vi "氨氮质控流程.vi"(7 "队列输入NH3":refnum<queue>, 10 "氨氮":bool, 11 "氨氮量程切换":enum32{"H", "L", "AUTO"}(ring)=enum."AUTO") -> (2 "氨氮中断报警":bool, 3 "布尔":bool)   [LabVIEW 2016, in "质控单元.lvlib"]
uses:
  <vilib>/ptbypt/NI_PtbyPt.lvlib
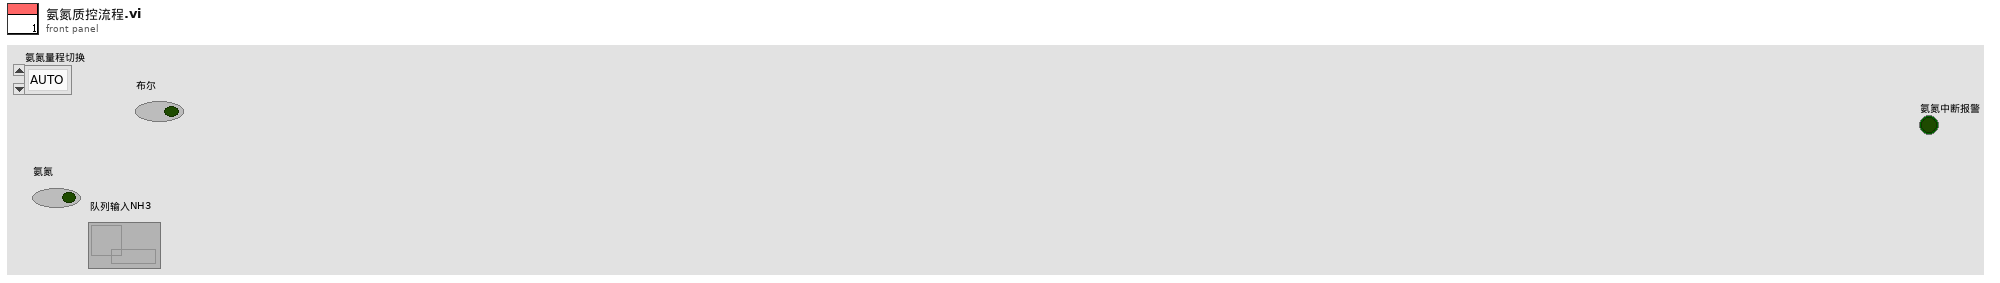
[diagram p1: front panel]
types:
  T1 = enum16{"待机", "启动氨氮水样", "氨氮测量中", "启动氨氮加标", "启动氨氮加标回收", "氨氮加标回收测量中", "启动总氮水样", "总氮测量中", "启动总氮加标", "启动总氮加标回收", "总氮加标回收测量中", "启动总磷水样", "总磷水样测量中", "启动总磷加标", "启动总磷加标回收", "总磷加标回收测量中", "结束"}
  T2 = cluster{"站号":u16, "量程切换":enum32{"H", "L", "AUTO"}, "控制命令":enum16{"启动测量", "标样核查", "零点核查", "跨度核查", "空白测试", "平行样测试", "加标回收", "空白校准", "标样校准", "初始化（清洗）", "停止测试", "仪器重启", "校时", "模式设置", "测量间隔设置"}, "模式设置":enum16{"待机", "连续模式", "周期模式", "定点模式", "受控模式", "手动模式"}, "测量间隔":u16}
  T3 = cluster{"时间标识":timestamp, "设备":string, "日志信息":string}
  T4 = cluster{"命令":string, cluster{"starting address":u16, "holding register value":u16}}
  T5 = cluster{"系统时间":timestamp, "工作状态":enum16{"空闲", "水样测试", "标样核查", "零点核查", "跨度核查", "空白测试", "平行样测试", "加标回收", "空白校准", "标样校准", "初始化（清洗）"}, "测量模式":enum16{"待机", "连续模式", "周期模式", "定点模式", "受控模式", "手动模式"}, "告警代码":enum16{"无告警", "缺试剂告警", "缺水样告警", "缺蒸馏水告警", "缺标液告警", "仪表漏液告警", "标定异常告警", "超量程告警", "加热异常", "低试剂预警", "超上限告警", "超下限告警", "仪表内部其他异常", "滴定异常告警", "电极异常告警", "量程切换告警", "参数设置告警", "PH电极电位异常", "电导率电极异常", "浊度光度异常", "溶解氧电极异常", "溶解氧光强异常", "温度异常告警", "PH异常告警", "溶解氧异常告警", "电导率异常告警", "浊度异常告警", "叶绿素异常告警", "藻密度异常告警", "蓝绿藻异常告警", "ORP异常告警", "氨氮异常告警", "清洁刷异常告警", "SD卡异常告警", "蓝牙异常告警", "Wifi异常告警", "流程异常告警"}, "故障代码":enum16{"无故障", "电机故障", "温度故障", "通讯故障", "滴定故障"}, "日志代码":u16, "软件版本":u16, "F0":sgl, "F1":sgl, "F2":sgl, "F3":sgl, "T":sgl, "H":sgl, "id":u16, "flowid":u16, "量程":u16, "总磷控温温度1":sgl, "营养盐控温温度2":sgl, "ADC":sgl}
  T6 = enum16{"空闲", "水样测试", "标样核查", "零点核查", "跨度核查", "空白测试", "平行样测试", "加标回收", "空白校准", "标样校准", "初始化（清洗）"}
  T7 = cluster{"因子编码":u32, "单位":u16, "标样参考值":sgl, "水样数据时间":timestamp, "水样实测值":sgl, "水样数据标识":string, "标样数据时间":timestamp, "标样实测值":sgl, "标样数据标识":string, "空白数据时间":timestamp, "空白实测值":sgl, "空白数据标识":string, "零点核查数据时间":timestamp, "零点核查实测值":sgl, "零点核查数据标识":string, "跨度核查数据时间":timestamp, "跨度核查实测值":sgl, "跨度核查数据标识":string, "加标回收数据时间":timestamp, "加标回收实测值":sgl, "加标回收数据标识":string, "平行样数据时间":timestamp, "平行样实测值":sgl, "平行样数据标识":string}
  T8 = cluster{"量程":dbl, "检出限":dbl, "加标前水样浓度":dbl, "加标后水样浓度":dbl, "加标水杯定容体积":dbl, "加标母液浓度":dbl, "加标体积":dbl, "加标回收率":dbl}
  T9 = cluster{"氨氮":u8, "总磷":u8, "总氮":u8, "CODMn":u8, "CODCr":u8}
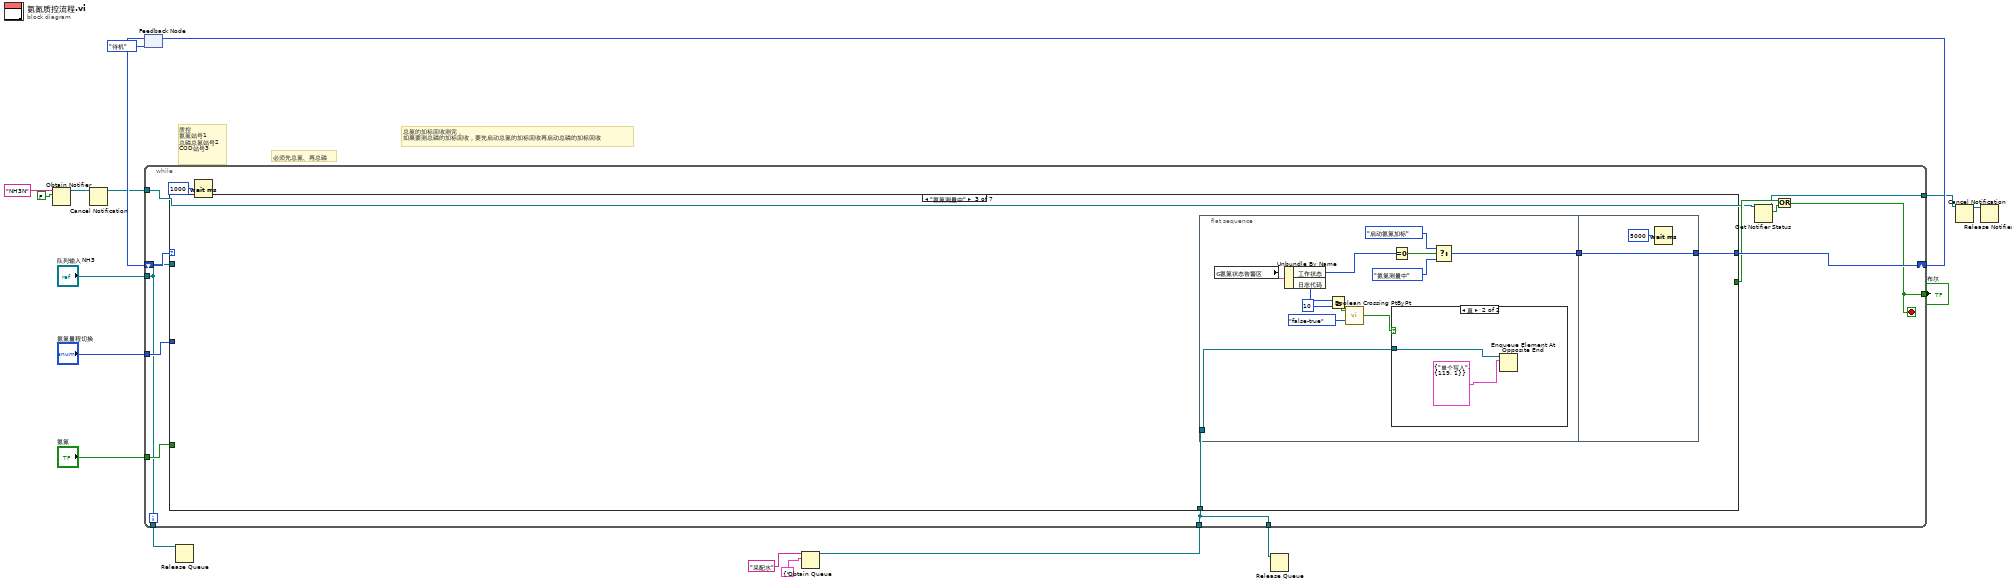
[diagram p0: block diagram]
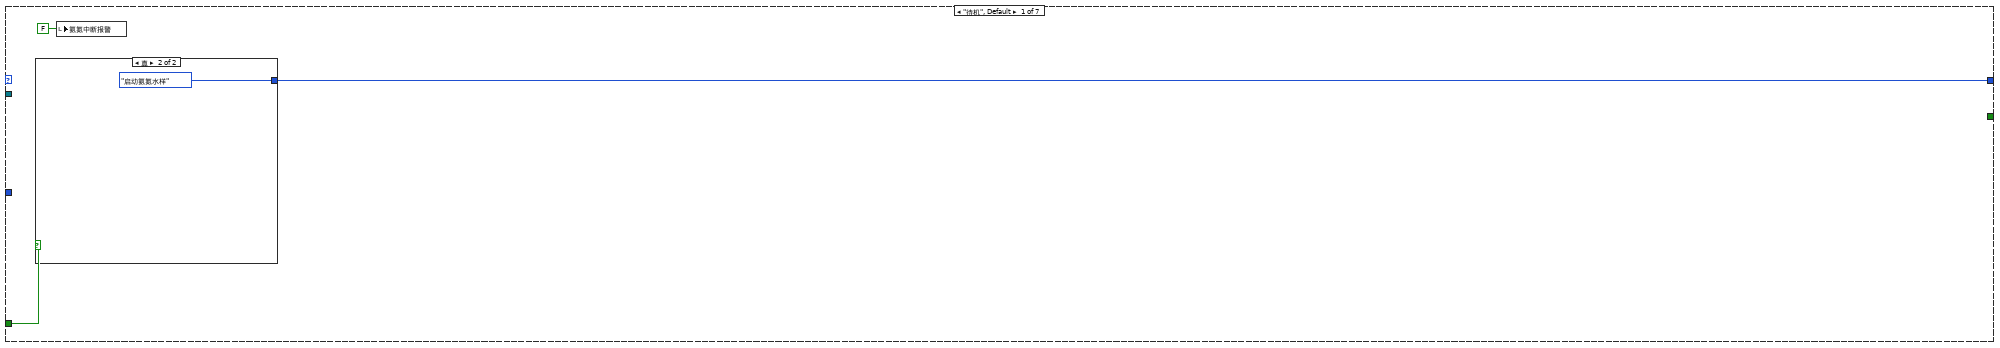
[diagram p2: hidden frame]
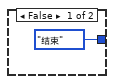
[diagram p3: hidden frame]
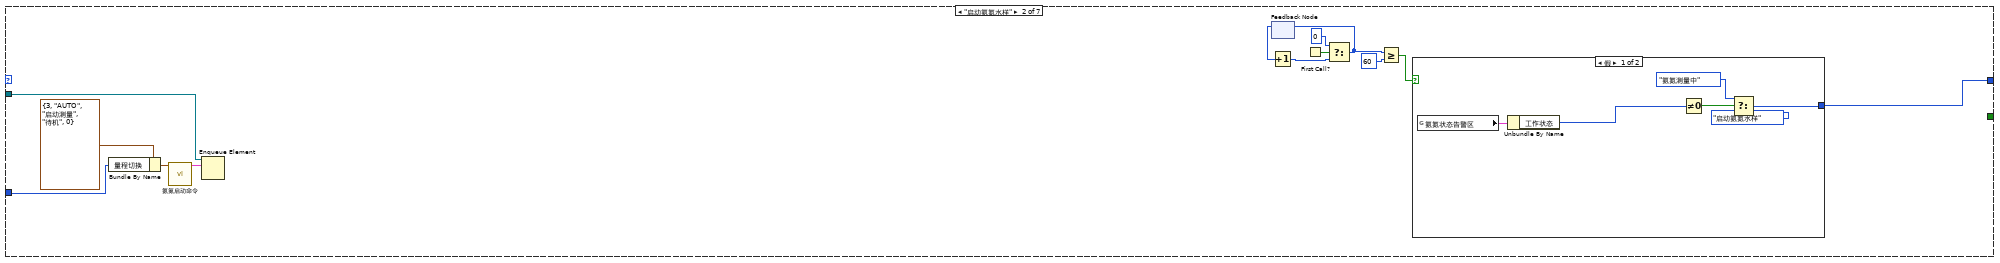
[diagram p4: hidden frame]
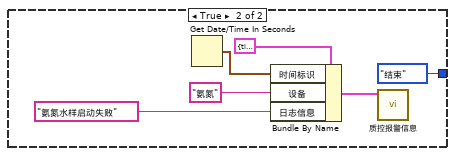
[diagram p5: hidden frame]
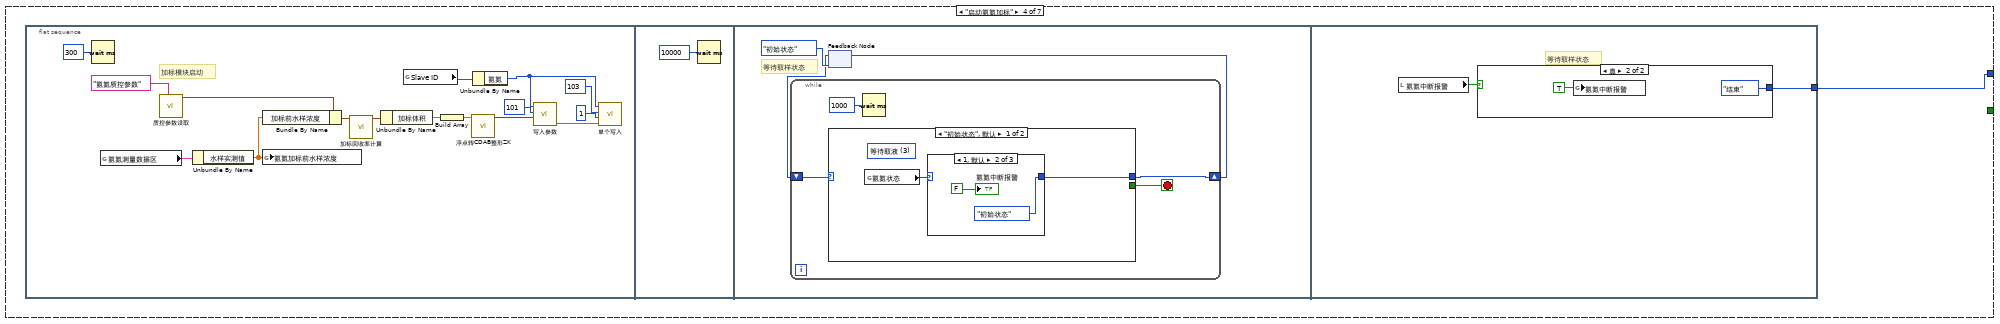
[diagram p7: hidden frame]
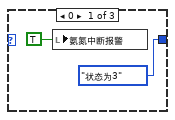
[diagram p8: hidden frame]
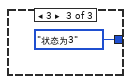
[diagram p9: hidden frame]
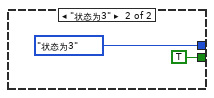
[diagram p10: hidden frame]
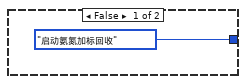
[diagram p11: hidden frame]
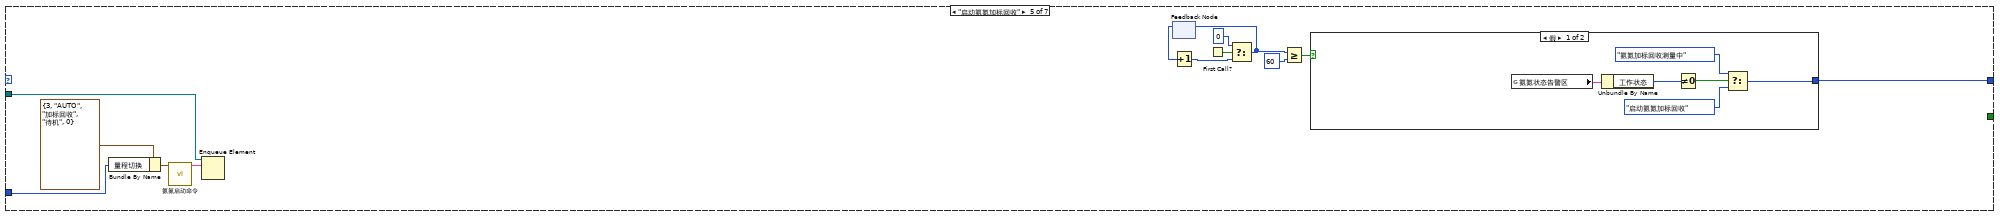
[diagram p12: hidden frame]
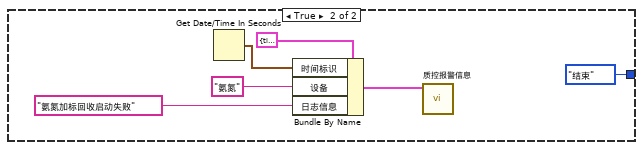
[diagram p13: hidden frame]
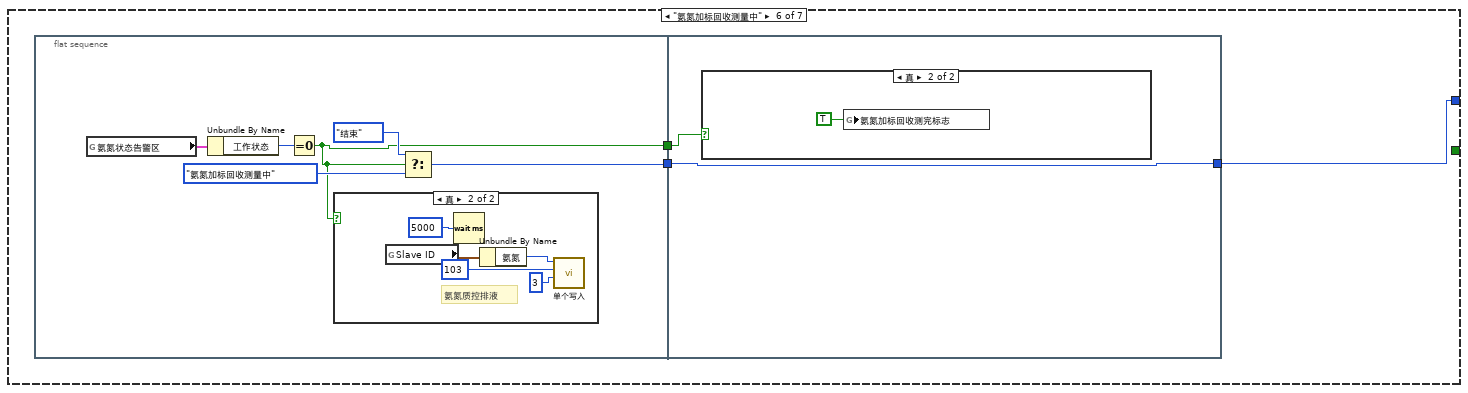
[diagram p14: hidden frame]
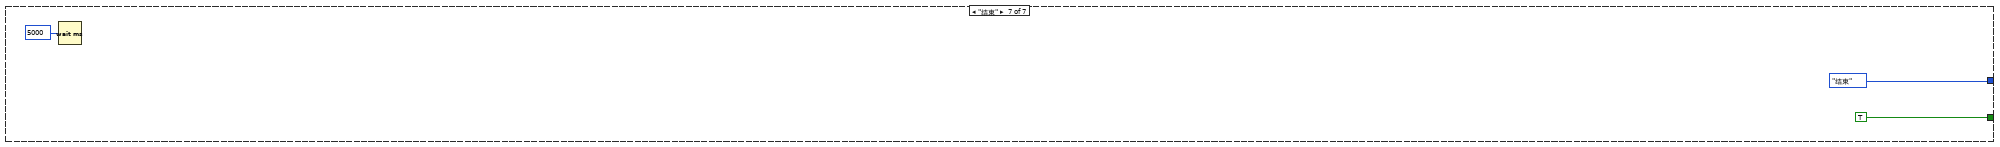
[diagram p17: hidden frame]
diagram:
  # "总氮的加标回收测完，\n如果要测总磷的加标回收，要先启动总氮的加标回收再启动总磷的加标回收"
  # "质控\n氨氮站号1   \n总磷总氮站号2\nCOD站号3"
  # "必须先总氮、再总磷"
  n1 = Obtain Notifier(name (unnamed)="NH3N" ("名称（未命名）"), notification data type=FALSE) -> (notifier out=w9:refnum<notifier>)  [unwired: 2 in, 2 out]
  n2 = Cancel Notification(0:w9) -> (8:w1:refnum<notifier>)  [unwired: 1 in, 2 out]
  n3 = feedback #1(T1."待机") -> (w12:T1)
  n4 = Obtain Queue(name (unnamed)="采配水" ("名称（未命名）"), element data type=cluster{"命令":string, "数据":variant} {"命令"="", "数据"=variant}) -> (queue out=w4:refnum<queue>)  [unwired: 3 in, 2 out]
  n5 = while {
    tunnel: "队列输入NH3" -> [w20]
    tunnel: "氨氮量程切换" -> [w28]
    tunnel: "氨氮" -> [w30]
    tunnel: [w23] -> w17
    shift-right: [w29] -> w15
    shift-left: w12 -> [w27]
    tunnel: w1 -> [w21]
    tunnel: [w22] -> w7
    tunnel: w4 -> [w19]
    tunnel: [w20] -> w3
    tunnel: [w19] -> w2
    stop <- w23 stop-if-true
    n6 = case shown="\"氨氮测量中\"" w27 {
      tunnel: [w33 w48 w63 w80 w124 w145 T1."结束"] -> w29
      tunnel: [_ _ _ _ _ _ TRUE] -> w24
      tunnel: w30 -> [w32 _ _ _ _ _ _]
      tunnel: w20 -> [_ w39 _ _ w122 _ _]
      tunnel: w28 -> [_ w36 _ _ w119 _ _]
      tunnel: w19 -> [_ _ w61 _ _ _ _]
      frame "待机", Default {
        n7 = case shown="真" w32 {
          tunnel: [T1."结束" T1."启动氨氮水样"] -> w33
          frame False {
          }
          frame True {
          }
        }
        n8 = local write "氨氮中断报警"(FALSE ("氨氮中断报警")) -> ()
      }
      frame "启动氨氮水样" {
        n9 = Bundle By Name(cluster=T2 {"站号"=3, "量程切换"=enum."AUTO", "控制命令"=enum."启动测量", "模式设置"=enum."待机", "测量间隔"=0} ("参数"), "量程切换"=w36) -> (w37:T2)
        n10 = call "氨氮启动命令.vi"("参数"=w37) -> ("启动命令"=w40:cluster{"命令":string, "data":variant})  [unwired: 10 in]
        n11 = Enqueue Element(queue=w39, element=w40) -> ()  [unwired: 2 in, 3 out]
        n12 = feedback #2() -> (w45:i32)  [unwired: 1 in]
        n13 = Increment(x=w45) -> (x+1=w44:i32)
        n14 = First Call?() -> (First Call?: T/F=w46:bool)
        n15 = Select(t=0, s=w46, f=w44) -> (s? t:f=w43:i32)
        n16 = feedback-in #2(w43) -> ()
        n17 = Greater Or Equal?(x=w43, y=60) -> (x >= y?=w41:bool)
        n18 = case shown="假" w41 {
          tunnel: [w52 T1."结束"] -> w48
          frame False {
            n19 = global read "与氨氮交互全局.vi" "氨氮状态告警区"() -> (w49:T5)
            n20 = Unbundle By Name(w49) -> ("工作状态"=w54:T6)
            n21 = Not Equal To 0?(x=w54) -> (x != 0?=w53:bool)
            n22 = Select(t=T1."氨氮测量中", s=w53, f=T1."启动氨氮水样") -> (s? t:f=w52:T1)
          }
          frame True {
            n23 = Get Date/Time In Seconds() -> (seconds since 1Jan1904=w60:timestamp)
            n24 = Bundle By Name(cluster=T3 {"时间标识"=timestamp(0 s since 1904-01-01), "设备"="", "日志信息"=""} ("data in"), "时间标识"=w60, "设备"="氨氮", "日志信息"="氨氮水样启动失败") -> (w55:T3)
            n25 = call "质控报警信息.vi"("data in"=w55) -> ()  [unwired: 11 in]
          }
        }
      }
      frame "氨氮测量中" {
        n26 = flat-sequence {
          tunnel: [w74] -> w62
          tunnel: w61 -> [w64]
          tunnel: [w79] -> w63
          tunnel: w62 -> [w79]
          frame #0 {
            n27 = global read "与氨氮交互全局.vi" "氨氮状态告警区"() -> (w70:T5)
            n28 = Unbundle By Name(w70) -> ("工作状态"=w75:T6, "日志代码"=w69:u16)
            n29 = Greater Or Equal?(x=w69, y=u16 10) -> (x >= y?=w67:bool)
            n30 = call <vilib>:"Boolean Crossing PtByPt.vi"("direction"=enum16{"either", "false-true", "true-false"}."false-true", "input"=w67) -> ("crossing"=w65:bool)  [unwired: 1 in]
            n31 = case shown="真" w65 {
              tunnel: w64 -> [_ w76]
              frame False {
              }
              frame True {
                n32 = Enqueue Element At Opposite End(queue=w76, element=T4 {"命令"="单个写入", {"starting address"=119, "holding register value"=1}} ("元素")) -> ()  [unwired: 2 in, 3 out]
              }
            }
            n33 = Equal To 0?(x=w75) -> (x = 0?=w73:bool)
            n34 = Select(t=T1."启动氨氮加标", s=w73, f=T1."氨氮测量中") -> (s? t:f=w74:T1)
          }
          frame #1 {
            n35 = Wait (ms)(milliseconds to wait=u32 5000 ("等待时间（毫秒）")) -> ()  [unwired: 1 out]
          }
        }
      }
      frame "启动氨氮加标" {
        n36 = flat-sequence {
          tunnel: [w115] -> w80
          frame #0 {
            # "加标模块启动"
            n37 = Wait (ms)(milliseconds to wait=u32 300 ("等待时间（毫秒）")) -> ()  [unwired: 1 out]
            n38 = global read "与氨氮交互全局.vi" "氨氮测量数据区"() -> (w84:T7)
            n39 = call "质控参数读取.vi"("section"="氨氮质控参数") -> ("参数"=w94:T8)  [unwired: 9 in, 1 out]
            n40 = Unbundle By Name(w84) -> ("水样实测值"=w85:sgl)
            n41 = Bundle By Name(cluster=w94, "加标前水样浓度"=w85) -> (w95:T8)
            n42 = global write "水样浓度全局.vi" "氨氮加标前水样浓度"(w85) -> ()
            n43 = call "加标回收率计算.vi"("参数"=w95) -> ("参数 out"=w93:T8)  [unwired: 9 in, 1 out]
            n44 = Unbundle By Name(w93) -> ("加标体积"=w86:dbl)
            n45 = global read "断电保存全局.vi" "Slave ID"() -> (w82:T9)
            n46 = Build Array(w86) -> (w92:dbl[])
            n47 = call "浮点转CDAB整形ZK.vi"("浮点数"=w92) -> ("CDAB整形输出"=w87:u16[])  [unwired: 10 in]
            n48 = Unbundle By Name(w82) -> ("氨氮"=w81:u8)
            n49 = call "写入参数.vi"("values"=w87, "starting address"=u16 101, "Slave ID"=w81) -> ("error out"=w91:errorcluster)  [unwired: 8 in]
            n50 = call "单个写入.vi"("Error in"=w91, "value"=u16 1, "address"=u16 103, "Slave ID"=w81) -> ()  [unwired: 7 in, 1 out]
          }
          frame #1 {
            n51 = Wait (ms)(milliseconds to wait=u32 10000 ("等待时间（毫秒）")) -> ()  [unwired: 1 out]
          }
          frame #2 {
            # "等待取样状态"
            n52 = feedback #3(enum16{"初始状态", "状态为3"}."初始状态") -> (w99:enum16{"初始状态", "状态为3"})
            n53 = while {
              shift-right: [w103] -> w98
              shift-left: w99 -> [w104]
              stop <- w102 stop-if-true
              n54 = case shown="\"初始状态\", 默认" w104 {
                tunnel: [w106 enum16{"初始状态", "状态为3"}."状态为3"] -> w103
                tunnel: [_ TRUE] -> w102
                frame "初始状态", Default {
                  (unwired) u16 3 items=["待机", "润洗", "进样", "等待取液", "排液"] ("氨氮状态")
                  n55 = global read "加标回收状态全局变量.vi" "氨氮状态"() -> (w105:u16)
                  n56 = case shown="1, 默认" w105 {
                    tunnel: [enum16{"初始状态", "状态为3"}."状态为3" enum16{"初始状态", "状态为3"}."初始状态" enum16{"初始状态", "状态为3"}."状态为3"] -> w106
                    frame 0 {
                      n57 = local write "氨氮中断报警"(TRUE ("氨氮中断报警")) -> ()
                    }
                    frame 1, Default {
                      "氨氮中断报警" <- FALSE ("总氮中断报警")
                    }
                    frame 3 {
                    }
                  }
                }
                frame "状态为3" {
                }
              }
              n58 = Wait (ms)(milliseconds to wait=u32 1000 ("等待时间（毫秒）")) -> ()  [unwired: 1 out]
            }
            n59 = feedback-in #3(w98) -> ()
          }
          frame #3 {
            # "等待取样状态"
            n60 = local read "氨氮中断报警"() -> (w114:bool)
            n61 = case shown="真" w114 {
              tunnel: [T1."启动氨氮加标回收" T1."结束"] -> w115
              frame False {
              }
              frame True {
                n62 = global write "质控中断报警全局.vi" "氨氮中断报警"(TRUE ("氨氮中断报警")) -> ()
              }
            }
          }
        }
      }
      frame "启动氨氮加标回收" {
        n63 = Bundle By Name(cluster=T2 {"站号"=3, "量程切换"=enum."AUTO", "控制命令"=enum."加标回收", "模式设置"=enum."待机", "测量间隔"=0} ("参数"), "量程切换"=w119) -> (w120:T2)
        n64 = call "氨氮启动命令.vi"("参数"=w120) -> ("启动命令"=w123:cluster{"命令":string, "data":variant})  [unwired: 10 in]
        n65 = Enqueue Element(queue=w122, element=w123) -> ()  [unwired: 2 in, 3 out]
        n66 = feedback #4() -> (w129:i32)  [unwired: 1 in]
        n67 = Increment(x=w129) -> (x+1=w128:i32)
        n68 = First Call?() -> (First Call?: T/F=w130:bool)
        n69 = Select(t=0, s=w130, f=w128) -> (s? t:f=w127:i32)
        n70 = feedback-in #4(w127) -> ()
        n71 = Greater Or Equal?(x=w127, y=60) -> (x >= y?=w125:bool)
        n72 = case shown="假" w125 {
          tunnel: [w135 T1."结束"] -> w124
          frame False {
            n73 = global read "与氨氮交互全局.vi" "氨氮状态告警区"() -> (w132:T5)
            n74 = Unbundle By Name(w132) -> ("工作状态"=w137:T6)
            n75 = Not Equal To 0?(x=w137) -> (x != 0?=w136:bool)
            n76 = Select(t=T1."氨氮加标回收测量中", s=w136, f=T1."启动氨氮加标回收") -> (s? t:f=w135:T1)
          }
          frame True {
            n77 = Get Date/Time In Seconds() -> (seconds since 1Jan1904=w143:timestamp)
            n78 = Bundle By Name(cluster=T3 {"时间标识"=timestamp(0 s since 1904-01-01), "设备"="", "日志信息"=""} ("data in"), "时间标识"=w143, "设备"="氨氮", "日志信息"="氨氮加标回收启动失败") -> (w138:T3)
            n79 = call "质控报警信息.vi"("data in"=w138) -> ()  [unwired: 11 in]
          }
        }
      }
      frame "氨氮加标回收测量中" {
        n80 = flat-sequence {
          tunnel: [w151] -> w146
          tunnel: [w147] -> w144
          tunnel: [w159] -> w145
          tunnel: w146 -> [w159]
          tunnel: w144 -> [w158]
          frame #0 {
            n81 = global read "与氨氮交互全局.vi" "氨氮状态告警区"() -> (w148:T5)
            n82 = Unbundle By Name(w148) -> ("工作状态"=w152:T6)
            n83 = Equal To 0?(x=w152) -> (x = 0?=w147:bool)
            n84 = case shown="真" w147 {
              frame False {
              }
              frame True {
                # "氨氮质控排液"
                n85 = global read "断电保存全局.vi" "Slave ID"() -> (w154:T9)
                n86 = Wait (ms)(milliseconds to wait=u32 5000 ("等待时间（毫秒）")) -> ()  [unwired: 1 out]
                n87 = Unbundle By Name(w154) -> ("氨氮"=w153:u8)
                n88 = call "单个写入.vi"("value"=u16 3, "address"=u16 103, "Slave ID"=w153) -> ()  [unwired: 8 in, 1 out]
              }
            }
            n89 = Select(t=T1."结束", s=w147, f=T1."氨氮加标回收测量中") -> (s? t:f=w151:T1)
          }
          frame #1 {
            n90 = case shown="真" w158 {
              frame False {
              }
              frame True {
                n91 = global write "质控测完标志全局 1.vi" "氨氮加标回收测完标志"(TRUE) -> ()
              }
            }
          }
        }
      }
      frame "结束" {
        n92 = Wait (ms)(milliseconds to wait=u32 5000 ("等待时间（毫秒）")) -> ()  [unwired: 1 out]
      }
    }
    n93 = Wait (ms)(milliseconds to wait=u32 1000 ("等待时间（毫秒）")) -> ()  [unwired: 1 out]
    n94 = Get Notifier Status(notifier=w21) -> (notifier out=w22:refnum<notifier>, current notification=w25:bool)  [unwired: 1 in, 3 out]
    n95 = Or(x=w24, y=w25) -> (x .or. y?=w23:bool)
  }
  "布尔" <- w17
  n96 = feedback-in #1(w15) -> ()
  n97 = Release Queue(queue=w3) -> ()  [unwired: 2 in, 3 out]
  n98 = Release Queue(queue=w2) -> ()  [unwired: 2 in, 3 out]
  n99 = Cancel Notification(0:w7) -> (8:w8:refnum<notifier>)  [unwired: 1 in, 2 out]
  n100 = Release Notifier(notifier=w8) -> ()  [unwired: 2 in, 3 out]
